vi "Abort all VIs.vi"() -> ()   [LabVIEW 2014]
panel:
  out "Array":path[](array[path])
  out "VI number":i32
  out "error out":errorcluster
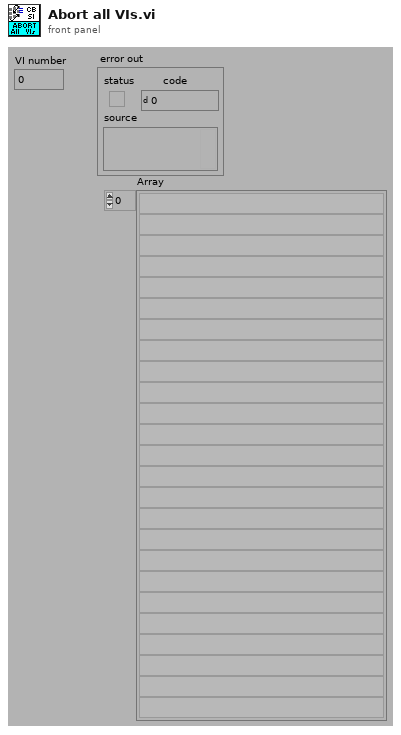
[diagram p1: front panel]
types:
  T1 = enum32{"Bad", "Idle", "Run top level", "Running"}
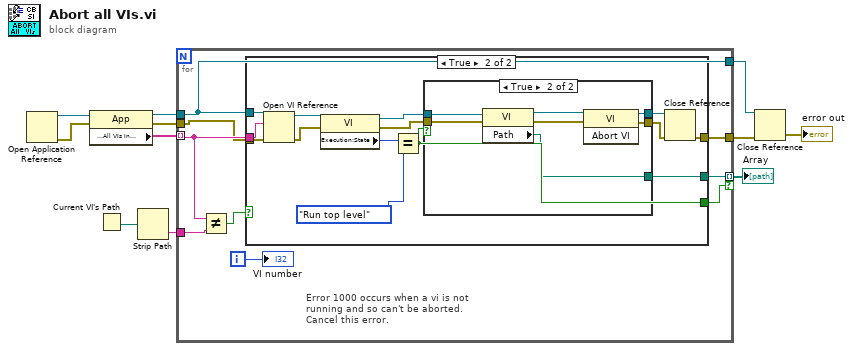
[diagram p0: block diagram]
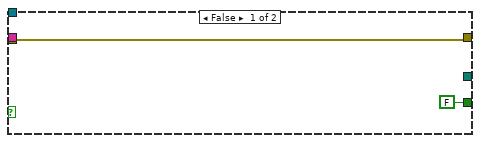
[diagram p2: hidden frame]
diagram:
  n1 = Open Application Reference() -> (0:w8:errorcluster, 3:w11:refnum<vi>)  [unwired: 1 in, 3 out]
  n2 = property class="App"(reference=w11, error in=w8) -> (reference out=w9:refnum<vi>, error out=w3:errorcluster, "Application:All VIs In Memory"=w10:string[])
  n3 = Current VI's Path() -> (path=w5:path)
  n4 = Strip Path(path=w5) -> (name=w4:string)  [unwired: 1 out]
  n5 = for {
    tunnel: w10 -> [w18] mode=indexing
    tunnel: w9 -> [w20]
    tunnel: [w20] -> w6
    tunnel: w4 -> [w17]
    tunnel: w3 -> [w15]
    tunnel: [w14] -> w2
    tunnel: [w13] -> w1 mode=indexing if=w12
    i -> [w19]
    # "Error 1000 occurs when a vi is not\nrunning and so can't be aborted.  \nCancel this error."
    n6 = Not Equal?(x=w18, y=w17) -> (x != y?=w16:bool)
    n7 = case shown="True" w16 {
      tunnel: w15 -> [w22 w34]
      tunnel: [w22 w33] -> w14
      tunnel: w20 -> [_ w32]
      tunnel: w18 -> [_ w31]
      tunnel: [_ w24] -> w13
      tunnel: [FALSE w23] -> w12
      frame False {
      }
      frame True {
        n8 = Open VI Reference(application reference (local)=w32, vi path=w31, error in (no error)=w34) -> (vi reference=w30:refnum<vi>, error out=w29:errorcluster)  [unwired: 3 out]
        n9 = property class="VI"(reference=w30, error in=w29) -> (reference out=w26:refnum<vi>, error out=w25:errorcluster, "Execution:State"=w28:T1)
        n10 = Equal?(x=w28, y=T1."Run top level" ("Execution:State")) -> (x = y?=w23:bool)
        n11 = case shown="True" w23 {
          tunnel: [w37 w45] -> w36
          tunnel: [w38 w44] -> w35
          tunnel: w26 -> [w38 w41]
          tunnel: w25 -> [w37 w43]
          tunnel: [_ w39] -> w24
          frame False {
          }
          frame True {
            n12 = property class="VI"(reference=w41, error in=w43) -> (reference out=w40:refnum<vi>, error out=w42:errorcluster, "Path"=w39:path)
            n13 = invoke class="VI" method="Abort VI"(reference=w40, error in=w42) -> (reference out=w44:refnum<vi>, error out=w45:errorcluster)  [unwired: 1 in, 1 out]
          }
        }
        n14 = Close Reference(reference=w35, error in (no error)=w36) -> (error out=w33:errorcluster)
      }
    }
    "VI number" <- w19
  }
  "Array" <- w1
  n15 = Close Reference(reference=w6, error in (no error)=w2) -> (error out=→"error out":errorcluster)
